vi "Buy Item.vi"(8 "error in (no error)":errorcluster, 11 "Items in":refnum<class "Items.lvclass">) -> (0 "error out":errorcluster, 3 "Items out":refnum<class "Items.lvclass">)   [LabVIEW 2020, in "Items.lvlib" / "Items.lvclass"]
uses:
  Items.lvclass
  Items.lvclass/Items.ctl
  <vilib>/ActorFramework/Actor/Actor.lvclass
  Controller Messages/Buy Product Msg/Buy Product Msg.lvclass
  C:/Program Files (x86)/National Instruments/LabVIEW 2020/vi.lib/ActorFramework/Actor/Actor.lvclass
  D:/Storage/Source Code/Clase AF/ClaseAF/13 Vending Machine/Items/Items.lvclass
  D:/Storage/Source Code/Clase AF/ClaseAF/13 Vending Machine/Panel Manager/Panel Manager.lvclass
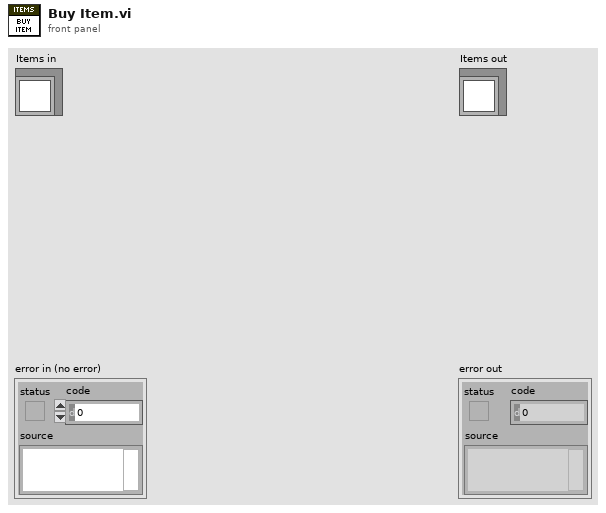
[diagram p1: front panel]
types:
  T1 = typedef "LVRowAndColumnTypeDef.ctl" = cluster{"Row":i32, "Column":i32}
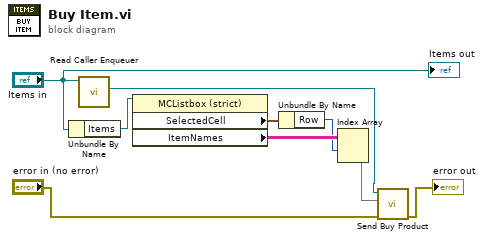
[diagram p0: block diagram]
diagram:
  n1 = Unbundle By Name("Items in") -> ("Items"=w9:refnum<vi>)
  n2 = call <vilib>:"Read Caller Enqueuer.vi"("Actor"="Items in") -> ("Caller Enqueuer"=w4:refnum<class "Message Enqueuer.lvclass">)  [unwired: 10 in]
  n3 = property class="MCListbox (strict)"(reference=w9) -> ("SelectedCell"=w7:T1, "ItemNames"=w8:string[][])  [unwired: 1 in, 2 out]
  n4 = Unbundle By Name(w7) -> ("Row"=w6:i32)
  n5 = Index Array(array=w8, index (row)=w6) -> (element=w3:string[])  [unwired: 1 in]
  n6 = call "Send Buy Product.vi"("error in (no error)"="error in (no error)", "Items"=w3, "Message Enqueuer"=w4) -> ("error out"=→"error out":errorcluster)  [unwired: 7 in, 1 out]
  "Items out" <- "Items in"
